vi "Send I8.vi"(7 "Priority":T1=enum."Normal" caption="Message Priority (Normal)", 8 "error in":errorcluster, 9 "I8":i8, 10 "_Message (I8) in":refnum<class "_Message (I8).lvclass">, 11 "Enqueuer":refnum<class "Message Enqueuer.lvclass">) -> (0 "error out":errorcluster, 3 "Message Enqueuer out":refnum<class "Message Enqueuer.lvclass">)   [LabVIEW 2014, in "MVC Subscription.lvlib" / "_Message (I8).lvclass"]
uses:
  _Message (I8).lvclass
  <vilib>/ActorFramework/Message Enqueuer/Message Priority.ctl
  <vilib>/ActorFramework/Message Enqueuer/Message Enqueuer.lvclass
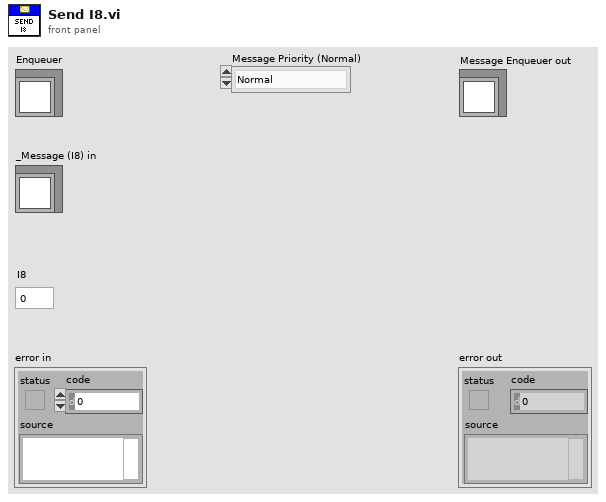
[diagram p1: front panel]
types:
  T1 = typedef "Actor Framework.lvlib/Message Enqueuer.lvclass/Message Priority.ctl" = enum16{"Low", "Normal", "High"}
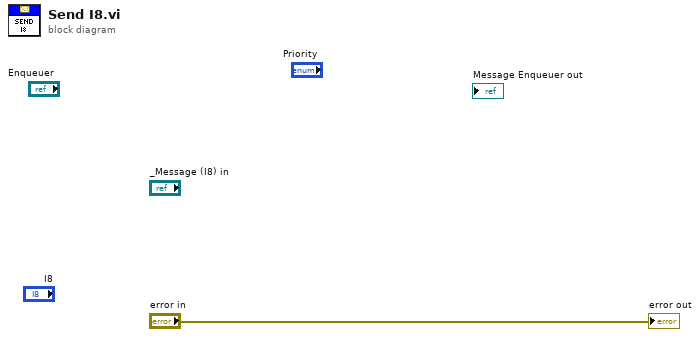
[diagram p0: block diagram]
diagram:
  "error out" <- "error in"
